vi "Check If Space Is Available in Sector Pixel FIFO.vi"() -> (3 "Space Avaliable?":bool)   [LabVIEW 2013]
uses:
  <vilib>/rvi/FIFO/Fifo_Resource/nirvififoEmulationSetSize.vi
  <vilib>/rvi/DataTransferAndStorage/Container/Common/niFpgaContainerGetUniqueNameForEmu.vi
  <vilib>/rvi/DataTransferAndStorage/Container/XNode/niFpgaContainer.xnode
  <vilib>/rvi/FIFO/Fifo_Resource/nirvififoEmulationGetNumberOfElementsToWrite.vi
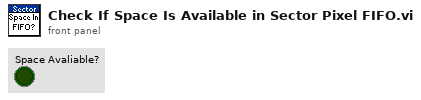
[diagram p1: front panel]
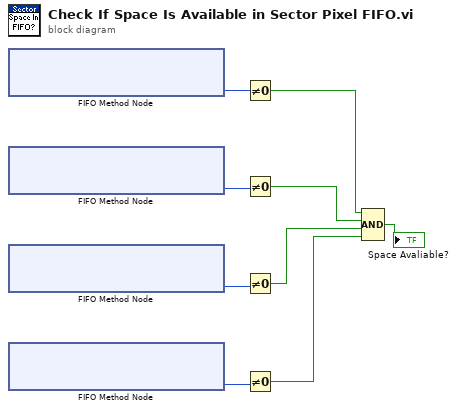
[diagram p0: block diagram]
diagram:
  n1 = xnode ("FIFO Method Node")() -> ("Number of Elements to Write"=w9:u32)  [unwired: 1 in, 1 out]
  n2 = xnode ("FIFO Method Node")() -> ("Number of Elements to Write"=w8:u32)  [unwired: 1 in, 1 out]
  n3 = xnode ("FIFO Method Node")() -> ("Number of Elements to Write"=w7:u32)  [unwired: 1 in, 1 out]
  n4 = xnode ("FIFO Method Node")() -> ("Number of Elements to Write"=w6:u32)  [unwired: 1 in, 1 out]
  n5 = Not Equal To 0?(x=w9) -> (x != 0?=w5:bool)
  n6 = Not Equal To 0?(x=w8) -> (x != 0?=w4:bool)
  n7 = Not Equal To 0?(x=w7) -> (x != 0?=w3:bool)
  n8 = Not Equal To 0?(x=w6) -> (x != 0?=w2:bool)
  n9 = Compound Arithmetic op=AND(w5, w4, w3, w2) -> (→"Space Avaliable?":bool)
